vi "table_v2.vi"(11 "Data":T1) -> (3 "array type (2D Dbl)":string[][](array[string]))   [LabVIEW 2022 SP3]
uses:
  controls/Data.ctl
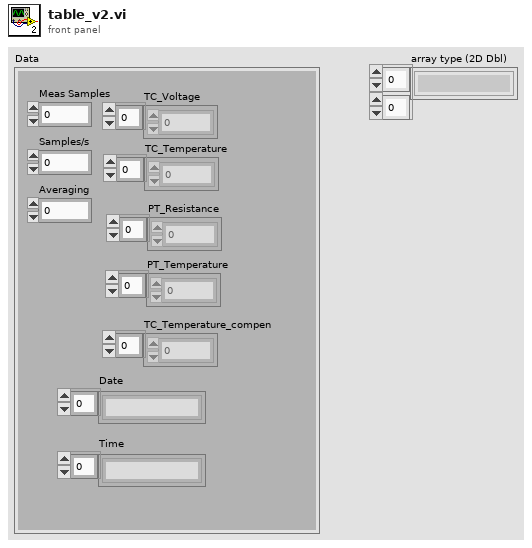
[diagram p1: front panel]
types:
  T1 = typedef "Data.ctl" = cluster{"Meas Samples":i32, "Samples/s":i32, "Averaging":i32, "TC_Voltage":dbl[], "TC_Temperature":dbl[], "PT_Resistance":dbl[], "PT_Temperature":dbl[], "TC_Temperature_compen":dbl[], "Date":string[], "Time":string[]}
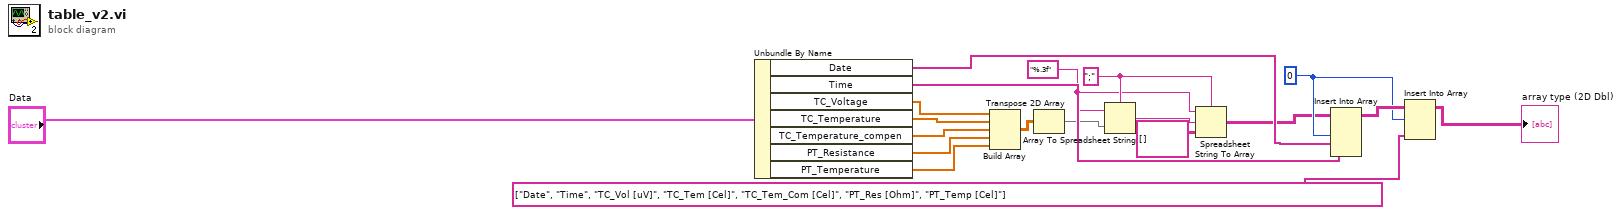
[diagram p0: block diagram]
diagram:
  w16 = 0 ("index (row)")
  w12 = ";" ("delimiter (Tab)")
  w11 = "%.3f" ("format string")
  n1 = Unbundle By Name("Data") -> ("Date"=w14:string[], "Time"=w15:string[], "TC_Voltage"=w6:dbl[], "TC_Temperature"=w1:dbl[], "TC_Temperature_compen"=w2:dbl[], "PT_Resistance"=w3:dbl[], "PT_Temperature"=w5:dbl[])
  n2 = Build Array(w6, w1, w2, w3, w5) -> (w4:dbl[][])
  n3 = Transpose 2D Array(2D array=w4) -> (transposed array=w8:dbl[][])
  n4 = Array To Spreadsheet String(delimiter (Tab)=w12, array=w8, 3:w11) -> (spreadsheet string=w9:string)
  n5 = Spreadsheet String To Array(delimiter (Tab)=w12, format string=w11, spreadsheet string=w9, array type (2D Dbl)=string[][] []) -> (array=w13:string[][])
  n6 = Insert Into Array(array=w13, index (col)=w16, new element #1=w14, new element #2=w15) -> (w18:string[][])  [unwired: 1 in]
  n7 = Insert Into Array(array=w18, index (row)=w16, new element=string[] ["Date", "Time", "TC_Vol [uV]", "TC_Tem [Cel]", "TC_Tem_Com [Cel]", "PT_Res [Ohm]", "PT_Temp [Cel]"]) -> (→"array type (2D Dbl)":string[][])  [unwired: 1 in]
